vi "Stop Core.vi"(10 "final error code":i32, 11 "Actor 1 - State machine in":refnum<class "Actor 1 - State machine.lvclass">) -> (3 "Actor 1 - State machine out":refnum<class "Actor 1 - State machine.lvclass">)   [LabVIEW 2020, in "Actor 1 - State machine.lvlib" / "Actor 1 - State machine.lvclass"]
doc: "(<B>Filename</B>: Actor Framework.lvlib:Actor.lvclass:Stop Core.vi)\n\nDefines what the actor does before it stops. Use the <B>final error code</B> input to determine whether the actor shut down in response to an error.\n\nBy default, this method passes the Stop message along to all auto-stop nested actors. A descendant class may override this method to define additional behavior, such as shutting down any processes the actor initiated in its override of the Actor Core method."
uses:
  Actor 1 - State machine.lvclass
  Actor 1 - State machine.lvclass/Actor 1 - State machine.ctl
  <vilib>/ActorFramework/Actor/Actor.lvclass
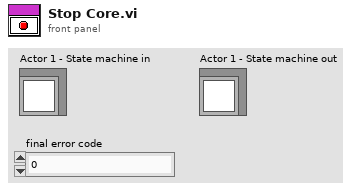
[diagram p1: front panel]
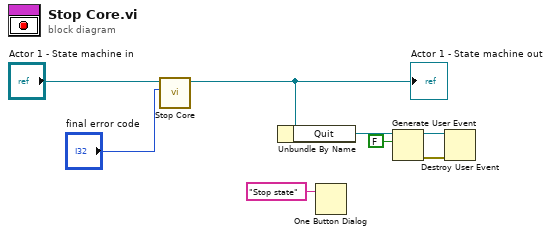
[diagram p0: block diagram]
diagram:
  n1 = call-parent "Stop Core.vi"("final error code"="final error code", "Actor in"="Actor 1 - State machine in") -> ("Actor out"=w4:refnum<class "Actor 1 - State machine.lvclass">)  [unwired: 9 in]
  "Actor 1 - State machine out" <- w4
  n2 = Unbundle By Name(w4) -> ("Quit"=w3:refnum<user-event>)
  n3 = One Button Dialog(message="Stop state") -> ()  [unwired: 1 in, 1 out]
  n4 = Generate User Event(user event=w3, event data cluster=FALSE ("event data")) -> (user event out=w5:refnum<user-event>, error out=w6:errorcluster)  [unwired: 2 in]
  n5 = Destroy User Event(user event=w5, error in=w6) -> ()  [unwired: 1 out]
